vi "Get Text Format Font String.vi"(8 "Error In":errorcluster, 9 "Font Name":string, 11 "Text Format Dialog":T4) -> (0 "Error Out":errorcluster, 3 "Text Format":T5 {"Font Size" min=6.0 step=1.0})   [LabVIEW 2021, in "Notebook.lvlib"]
uses:
  Notebook.lvlib
  Rich Text Box/Text Formatting.ctl
  Rich Text Box/Text Colors.ctl
  Rich Text Box/Text Style.ctl
  Rich Text Box/Text Alignment.ctl
  Rich Text Box/Rich Text Box.lvlib
panel:
  # "see the License on the block diagram (Ctrl+E or Window:Show Block Diagram)"
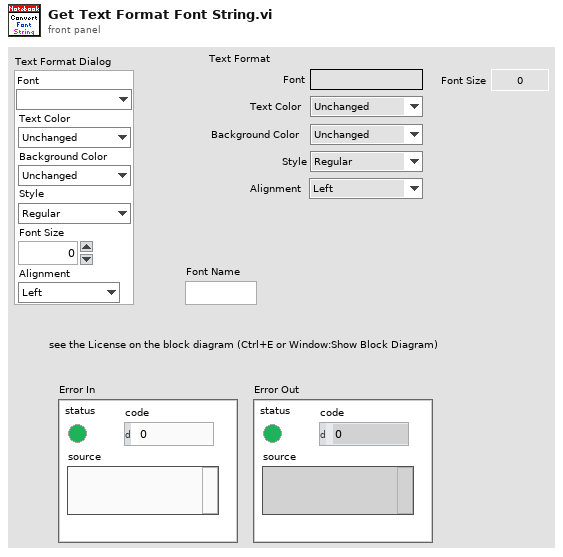
[diagram p1: front panel]
types:
  T1 = typedef "Rich Text Box.lvlib/Text Colors.ctl" = enum16{"Unchanged", "Black", "Blue", "Cyan", "Maroon", "Gray", "Violet", "Green", "Light Green", "Orange", "Yellow", "Magenta", "Red", "White"}
  T2 = typedef "Rich Text Box.lvlib/Text Style.ctl" = enum16{"Regular", "Bold", "Italic", "Underline", "Strikeout"}
  T3 = typedef "Rich Text Box.lvlib/Text Alignment.ctl" = enum16{"Left", "Right", "Center"}
  T4 = cluster{"Font":u16, "Text Color":T1, "Background Color":T1, "Style":T2, "Font Size":dbl, "Alignment":T3}
  T5 = typedef "Rich Text Box.lvlib/Text Formatting.ctl" = cluster{"Font":string, "Text Color":T1, "Background Color":T1, "Style":T2, "Font Size":dbl, "Alignment":T3}
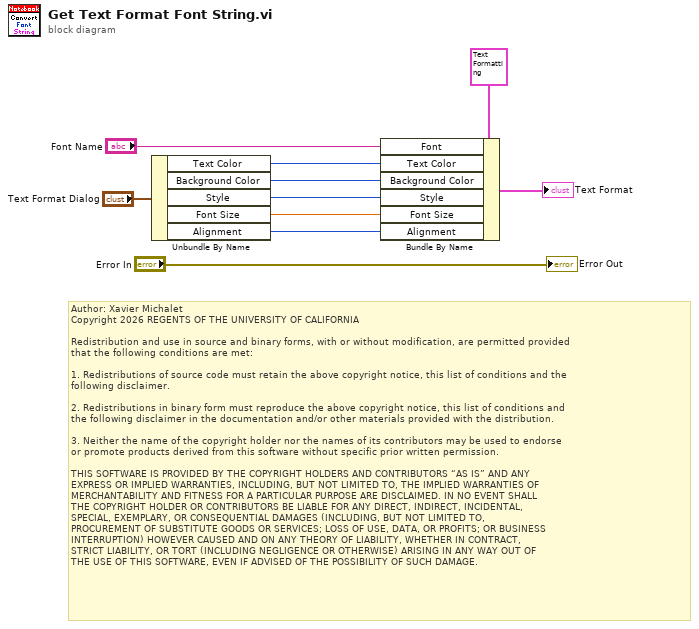
[diagram p0: block diagram]
diagram:
  # "Author: Xavier Michalet\nCopyright 2026 REGENTS OF THE UNIVERSITY OF CALIFORNIA\n\nRedistribution and use in source and binary forms, with or without modification, are permitted provided\nthat the following conditions are met:\n\n1. Redistributions of source code must retain the above copyright notice, this list of conditions and the\nfollowing disclaimer.\n\n2. Redistributions in binary form must reproduce the above copyright notice, this list of conditions and\nthe following disclaimer in the documentation and/or other materials provided with the distribution.\n\n3. Neither the name of the copyright holder nor the names of its contributors may be used to endorse \nor promote products derived from this software without specific prior written permission.\n\nTHIS SOFTWARE IS PROVIDED BY THE COPYRIGHT HOLDERS AND CONTRIBUTORS “AS IS” AND ANY \nEXPRESS OR IMPLIED WARRANTIES, INCLUDING, BUT NOT LIMITED TO, THE IMPLIED WARRANTIES OF\nMERCHANTABILITY AND FITNESS FOR A PARTICULAR PURPOSE ARE DISCLAIMED. IN NO EVENT SHALL\nTHE COPYRIGHT HOLDER OR CONTRIBUTORS BE LIABLE FOR ANY DIRECT, INDIRECT, INCIDENTAL, \nSPECIAL, EXEMPLARY, OR CONSEQUENTIAL DAMAGES (INCLUDING, BUT NOT LIMITED TO, \nPROCUREMENT OF SUBSTITUTE GOODS OR SERVICES; LOSS OF USE, DATA, OR PROFITS; OR BUSINESS\nINTERRUPTION) HOWEVER CAUSED AND ON ANY THEORY OF LIABILITY, WHETHER IN CONTRACT, \nSTRICT LIABILITY, OR TORT (INCLUDING NEGLIGENCE OR OTHERWISE) ARISING IN ANY WAY OUT OF\nTHE USE OF THIS SOFTWARE, EVEN IF ADVISED OF THE POSSIBILITY OF SUCH DAMAGE."
  n1 = Unbundle By Name("Text Format Dialog") -> ("Text Color"=w6:T1, "Background Color"=w5:T1, "Style"=w2:T2, "Font Size"=w4:dbl, "Alignment"=w3:T3)
  n2 = Bundle By Name(cluster=T5 {"Font"="", "Text Color"=enum."Unchanged", "Background Color"=enum."Unchanged", "Style"=enum."Regular", "Font Size"=-1.0, "Alignment"=enum."Left"} ("Text Formatting"), "Font"="Font Name", "Text Color"=w6, "Background Color"=w5, "Style"=w2, "Font Size"=w4, "Alignment"=w3) -> (→"Text Format":T5)
  "Error Out" <- "Error In"
